vi "tlc_Play.vi"(7 "Reset":bool, 8 "error in (no error)":errorcluster) -> (0 "error out":errorcluster, 3 "Stop?":bool)   [LabVIEW 2010]
doc: "This VI will perform the functionality for playing a Cue for the Theatre Light Controller."
uses:
  Controls/Play.ctl
  Controls/Cue State.ctl
  Modules/Cue/tlc_Cue_Information Command.ctl
  Controls/tlc_User Interface Data Type.ctl
  Modules/Timing/tlc_Timing Command Control.ctl
panel:
  # "Input Data"
  # "Internal Data"
  # "Output Data"
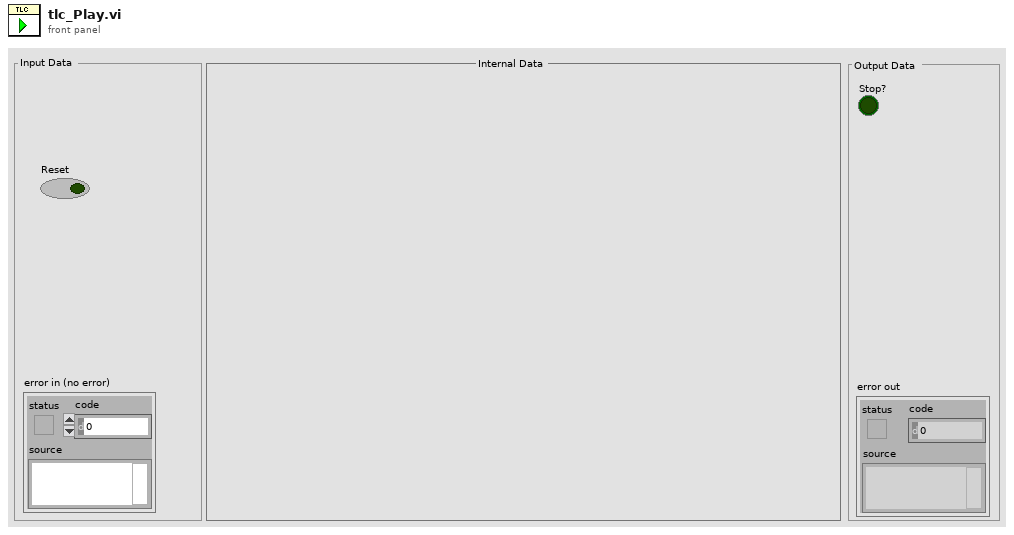
[diagram p1: front panel]
types:
  T1 = typedef "Play.ctl" = enum16{"Initialize", "Begin Play", "Load Cue", "Wait Time", "Fade Time", "Follow Time", "Check for Next Cue", "End Play"}
  T2 = typedef "tlc_Timing Command Control.ctl" = enum16{"Start", "Check Time"}
  T3 = typedef "Cue State.ctl" = cluster{"Desired Intensity":dbl, "Desired Color":u32}
  T4 = typedef "tlc_Cue_Information Command.ctl" = enum16{"Add Cue", "Get Cue Values", "Set Cue Values", "Get Number of Cues", "Initialize", "Get Empty Cue"}
  T5 = typedef "tlc_Cue_Information.ctl" = cluster{"Cue Name":string, "Wait Time (s)":u32, "Fade Time (s)":u32, "Follow Time (s)":u32, "Channels":T6[][]}
  T6 = typedef "channel.ctl" = cluster{"Intensität":dbl, " Farbe":u32, "Channel":i32}
  T7 = typedef "tlc_User Interface Data Type.ctl" = enum16{"Initialize", "Initialize Front Panel", "Update Front Panel Channels", "Select Cue in Cue List", "Enable/Disable Front Panel Controls", "Update Cue List", "Stop"}
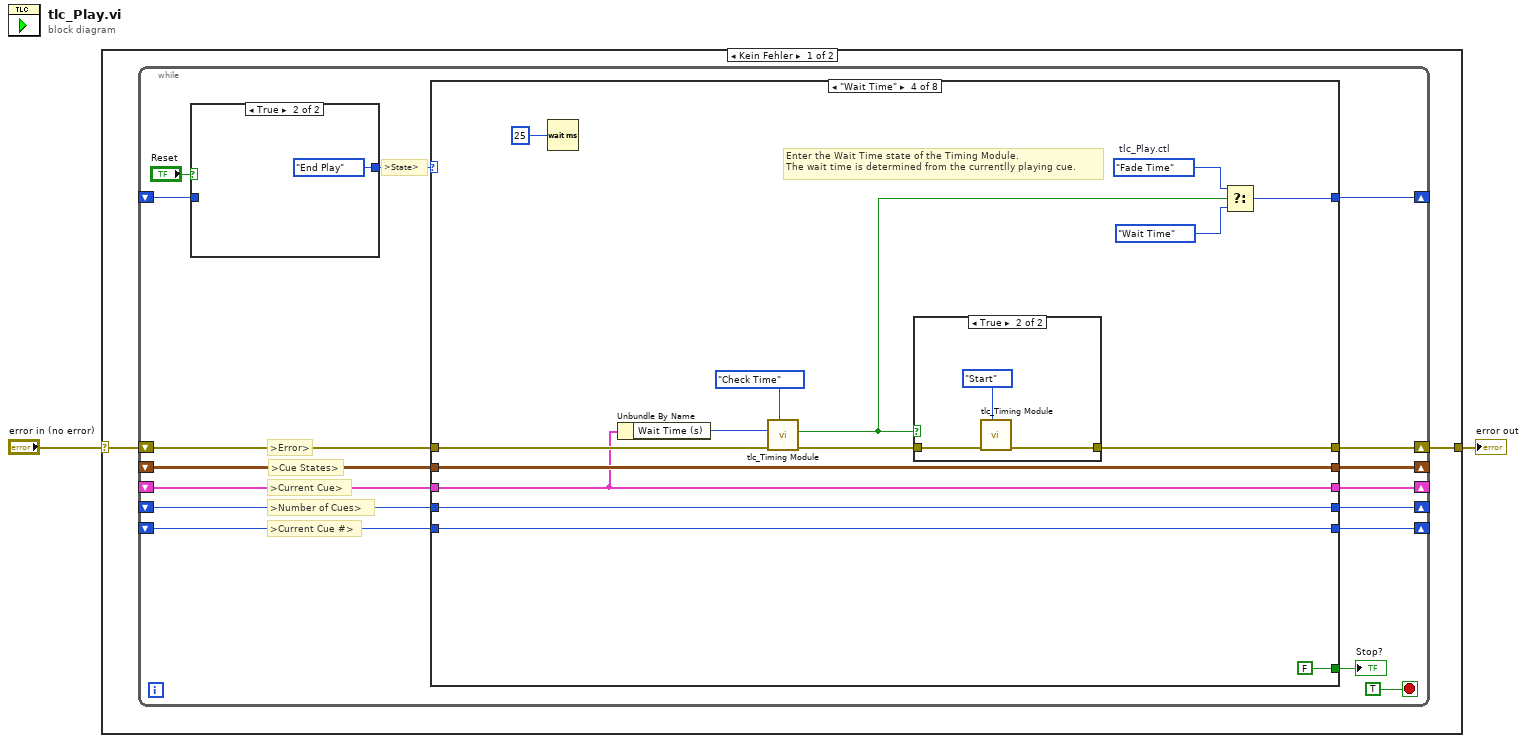
[diagram p0: block diagram]
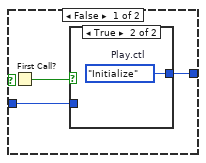
[diagram p2: hidden frame]
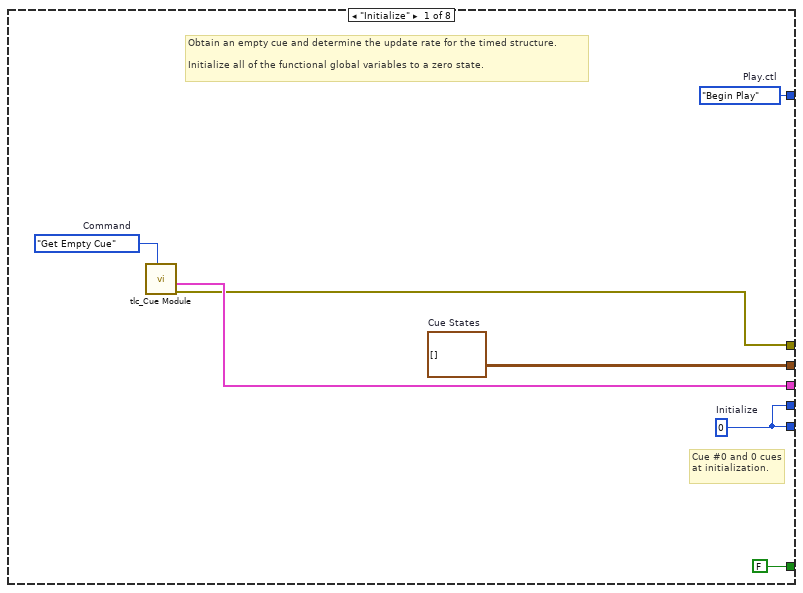
[diagram p4: hidden frame]
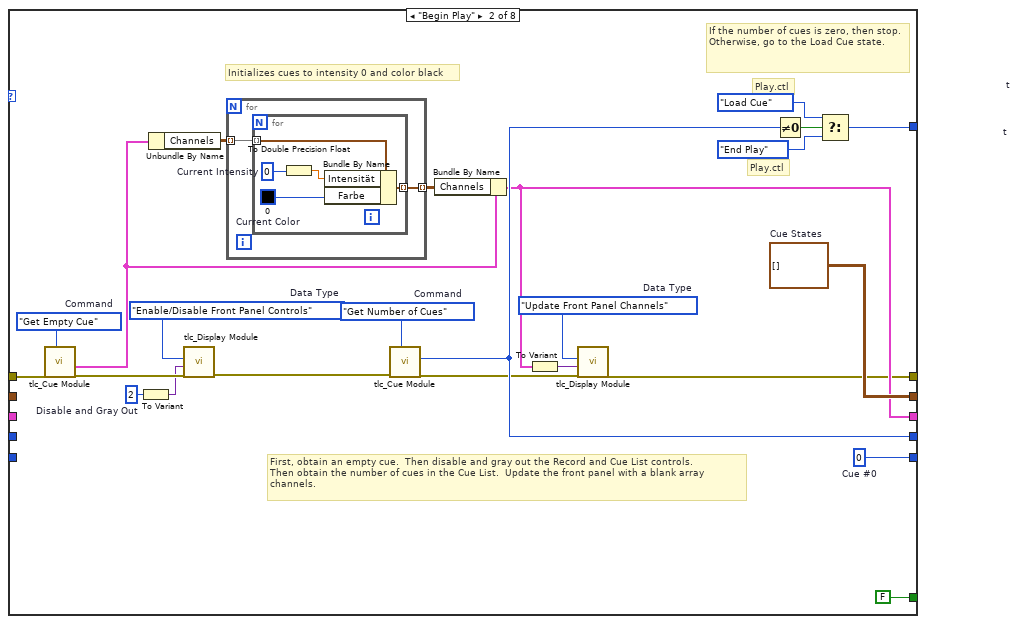
[diagram p5: hidden frame]
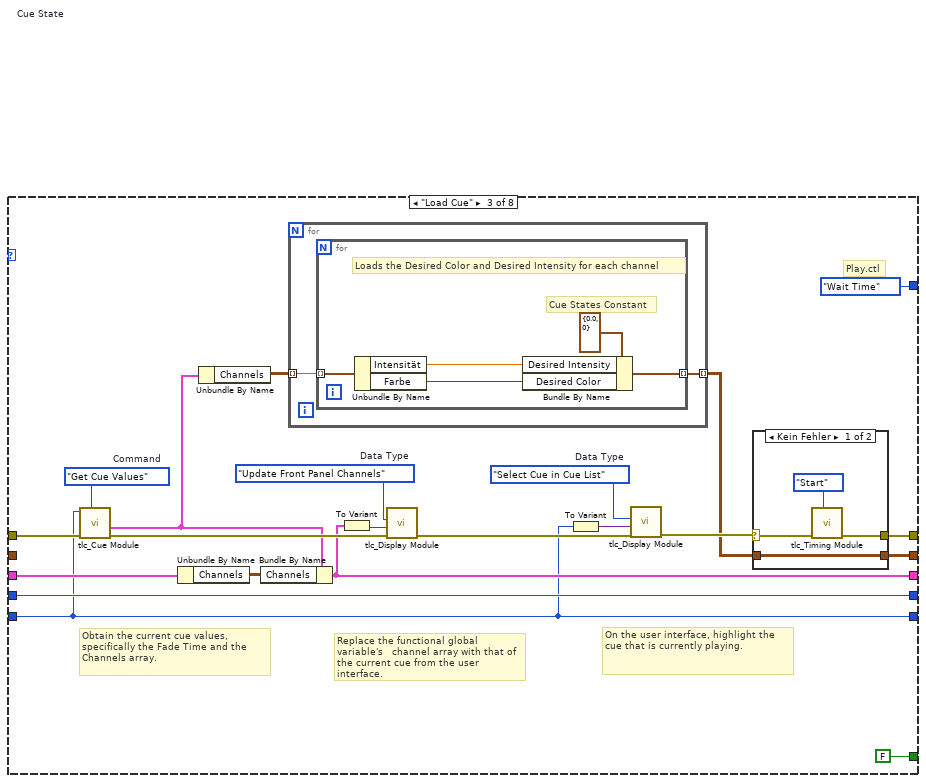
[diagram p6: hidden frame]
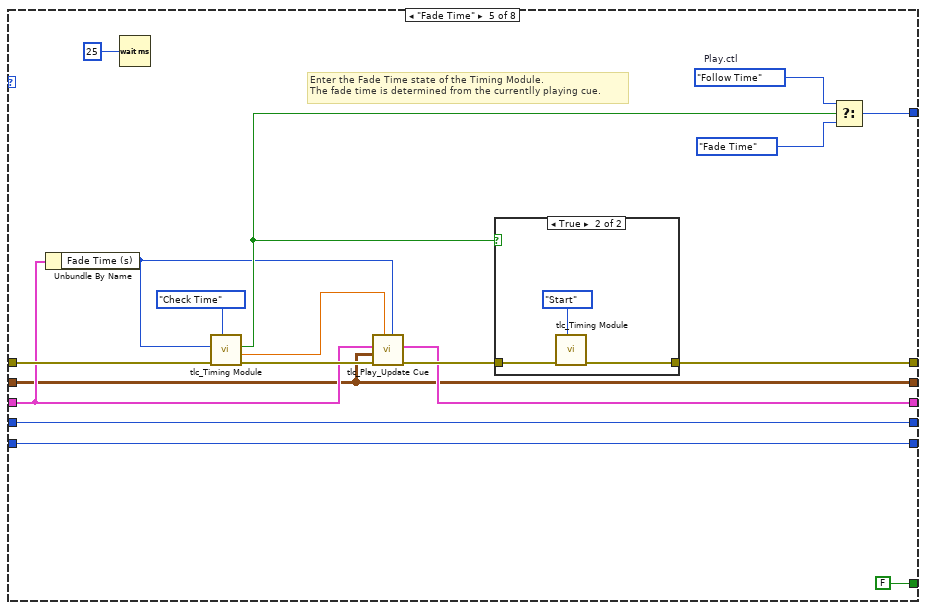
[diagram p9: hidden frame]
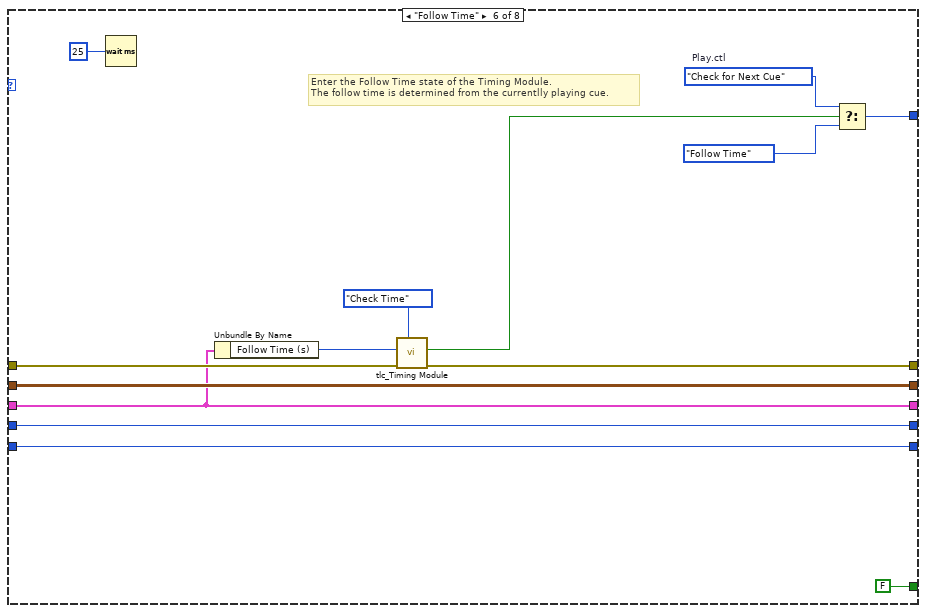
[diagram p11: hidden frame]
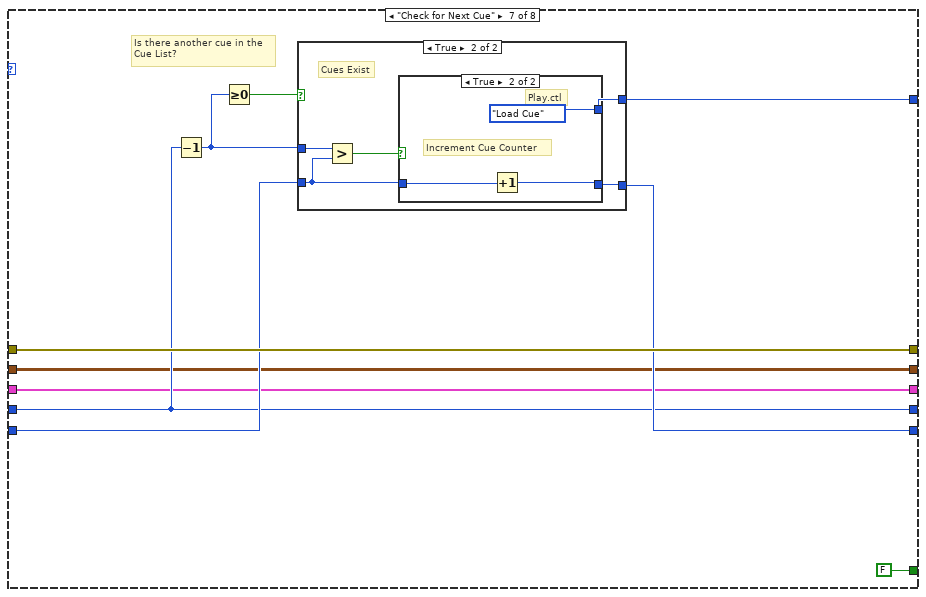
[diagram p12: hidden frame]
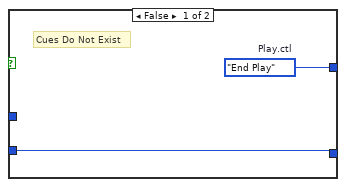
[diagram p13: hidden frame]
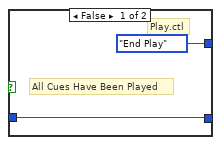
[diagram p14: hidden frame]
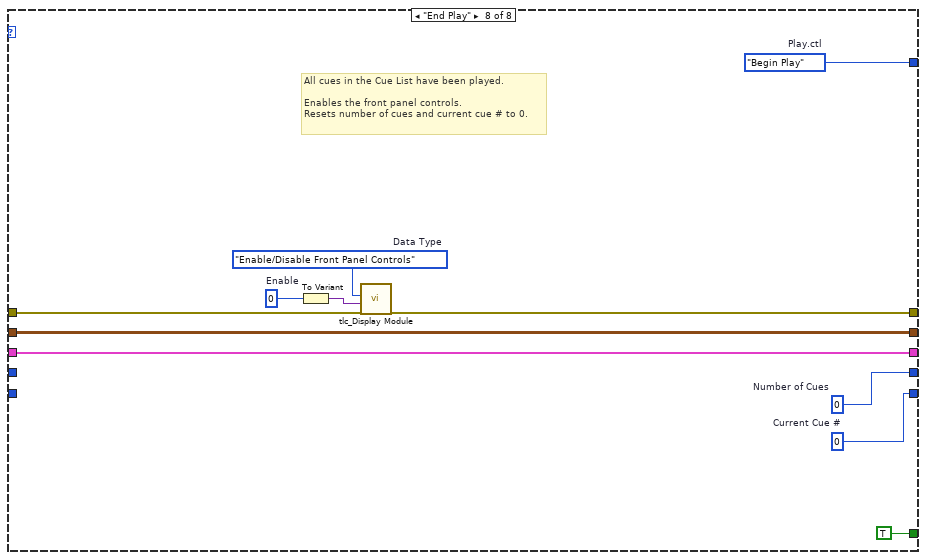
[diagram p15: hidden frame]
diagram:
  n1 = case shown="Kein Fehler" "error in (no error)" {
    selector: "error in (no error)" -> [w3 w187]
    tunnel: [w4 w187] -> w2
    frame No Error {
      n2 = while {
        shift-right: [w19] -> _
        shift-left: _ -> [w8]
        shift-right: [w12] -> w4
        shift-left: w3 -> [w20]
        shift-right: [w18] -> _
        shift-left: _ -> [w17]
        shift-right: [w13] -> _
        shift-left: _ -> [w16]
        shift-right: [w14] -> _
        shift-left: _ -> [w15]
        shift-right: [w7] -> _
        shift-left: _ -> [w6]
        stop <- TRUE stop-if-true
        # ">Cue States>"
        # ">Error>"
        # ">Current Cue #>"
        # ">Number of Cues>"
        # ">State>"
        # ">Current Cue>"
        n3 = case shown="True" "Reset" {
          tunnel: [w23 Play."End Play" ("Play.ctl")] -> w9
          tunnel: w8 -> [w22 _]
          frame False {
            n4 = First Call?() -> (First Call?: T/F=w21:bool)
            n5 = case shown="True" w21 {
              tunnel: [w24 w25] -> w23
              tunnel: w22 -> [w24 _]
              frame False {
              }
              frame True {
                w25 = Play."Initialize"  # Play.ctl
              }
            }
          }
          frame True {
          }
        }
        n6 = case shown="\"Wait Time\"" w9 {
          tunnel: [FALSE FALSE FALSE FALSE FALSE FALSE FALSE TRUE] -> w10
          tunnel: w20 -> [_ w44 w80 w109 w130 w149 w163 w176]
          tunnel: [w27 w34 w67 w104 w132 w145 w163 w180] -> w12
          tunnel: [w32 w54 Play."Wait Time" w103 w128 w144 w160 w186] -> w19
          tunnel: [w33 w45 w73 w113 w135 w153 w156 w183] -> w18
          tunnel: w17 -> [_ _ w73 w113 w135 w153 w156 _]
          tunnel: [w30 w38 w71 w107 w119 w147 w155 w184] -> w13
          tunnel: w16 -> [_ _ w82 w107 w120 w147 w155 w184]
          tunnel: w15 -> [_ _ w70 w112 w134 w152 w158 _]
          tunnel: [w33 w53 w70 w112 w134 w152 w161 w182] -> w14
          tunnel: [w28 w39 w66 w110 w118 w150 w154 w181] -> w7
          tunnel: w6 -> [_ _ _ w110 w118 w150 w154 w181]
          frame "Initialize" {
            w28 = T3[][] []  # Cue States
            w29 = tlc_Cue_Information_Command."Get Empty Cue"  # Command
            w32 = Play."Begin Play"  # Play.ctl
            w33 = 0  # Initialize
            # "Obtain an empty cue and determine the update rate for the timed structure.\n\nInitialize all of the functional global variables to a zero state."
            # "Cue #0 and 0 cues at initialization."
            n7 = call "tlc_Cue Module.vi"("Command"=w29) -> ("error out"=w27:errorcluster, "Cue Output"=w30:T5)  [unwired: 7 in, 1 out]
          }
          frame "Begin Play" {
            w39 = T3[][] []  # Cue States
            w40 = tlc_User_Interface_Data_Type."Update Front Panel Channels"  # Data Type
            w46 = tlc_Cue_Information_Command."Get Number of Cues"  # Command
            w47 = tlc_User_Interface_Data_Type."Enable/Disable Front Panel Controls"  # Data Type
            w48 = tlc_Cue_Information_Command."Get Empty Cue"  # Command
            w55 = Play."End Play"  # t
            w56 = Play."Load Cue"  # t
            w36 = 2  # Disable and Gray Out
            w53 = 0  # Cue #0
            # "Initializes cues to intensity 0 and color black"
            # "If the number of cues is zero, then stop.\nOtherwise, go to the Load Cue state."
            # "First, obtain an empty cue.  Then disable and gray out the Record and Cue List controls.\nThen obtain the number of cues in the Cue List.  Update the front panel with a blank array \nchannels."
            # "Play.ctl"
            # "Play.ctl"
            n8 = call "tlc_Cue Module.vi"("Command"=w48, "error in (no error)"=w44) -> ("error out"=w43:errorcluster, "Cue Output"=w49:T5)  [unwired: 6 in, 1 out]
            n9 = To Variant(anything=w36) -> (Variant=w35:variant)
            n10 = Unbundle By Name(w49) -> ("Channels"=w52:T6[][])
            n11 = call "tlc_Display Module.vi"("error in (no error)"=w43, "Data"=w35, "Data Type"=w47) -> ("error out"=w42:errorcluster)  [unwired: 8 in]
            n12 = for {
              tunnel: w52 -> [w59] mode=indexing
              tunnel: [w58] -> w51 mode=indexing
              n13 = for {
                tunnel: w59 -> [w64] mode=indexing
                tunnel: [w62] -> w58 mode=indexing
                w63 = u32 0  # Current Color
                w61 = u32 0  # Current Intensity
                n14 = To Double Precision Float(number=w61) -> (double precision float=w60:dbl)
                n15 = Bundle By Name(cluster=w64, "Intensität"=w60, "Farbe"=w63) -> (w62:T6)
              }
            }
            n16 = call "tlc_Cue Module.vi"("Command"=w46, "error in (no error)"=w42) -> ("error out"=w41:errorcluster, "Number of Cues"=w45:i32)  [unwired: 6 in, 1 out]
            n17 = Bundle By Name(cluster=w49, "Channels"=w51) -> (w38:T5)
            n18 = To Variant(anything=w38) -> (Variant=w37:variant)
            n19 = call "tlc_Display Module.vi"("error in (no error)"=w41, "Data"=w37, "Data Type"=w40) -> ("error out"=w34:errorcluster)  [unwired: 8 in]
            n20 = Not Equal To 0?(x=w45) -> (x != 0?=w57:bool)
            n21 = Select(t=w56, s=w57, f=w55) -> (s? t:f=w54:T1)
          }
          frame "Load Cue" {
            w74 = tlc_User_Interface_Data_Type."Select Cue in Cue List"  # Data Type
            w76 = tlc_User_Interface_Data_Type."Update Front Panel Channels"  # Data Type
            w78 = tlc_Cue_Information_Command."Get Cue Values"  # Command
            # "On the user interface, highlight the cue that is currently playing."
            # "Replace the functional global variable's   channel array with that of the current cue from the user interface."
            # "Obtain the current cue values, specifically the Fade Time and the Channels array."
            # "Play.ctl"
            n22 = call "tlc_Cue Module.vi"("Command"=w78, "error in (no error)"=w80, "Cue Index"=w70) -> ("error out"=w79:errorcluster, "Cue Output"=w77:T5)  [unwired: 5 in, 1 out]
            n23 = Unbundle By Name(w82) -> ("Channels"=w81:T6[][])
            n24 = Unbundle By Name(w77) -> ("Channels"=w84:T6[][])
            n25 = Bundle By Name(cluster=w77, "Channels"=w81) -> (w71:T5)
            n26 = for {
              tunnel: w84 -> [w93] mode=indexing
              tunnel: [w92] -> w65 mode=indexing
              n27 = for {
                tunnel: w93 -> [w98] mode=indexing
                tunnel: [w96] -> w92 mode=indexing
                w95 = T3 {"Desired Intensity"=0.0, "Desired Color"=0}  # Cue State
                # "Loads the Desired Color and Desired Intensity for each channel"
                # "Cue States Constant"
                n28 = Unbundle By Name(w98) -> ("Intensität"=w94:dbl, "Farbe"=w97:u32)
                n29 = Bundle By Name(cluster=w95, "Desired Intensity"=w94, "Desired Color"=w97) -> (w96:T3)
              }
            }
            n30 = To Variant(anything=w71) -> (Variant=w72:variant)
            n31 = call "tlc_Display Module.vi"("error in (no error)"=w79, "Data"=w72, "Data Type"=w76) -> ("error out"=w75:errorcluster)  [unwired: 8 in]
            n32 = To Variant(anything=w70) -> (Variant=w69:variant)
            n33 = call "tlc_Display Module.vi"("error in (no error)"=w75, "Data"=w69, "Data Type"=w74) -> ("error out"=w68:errorcluster)  [unwired: 8 in]
            n34 = case shown="Kein Fehler" w68 {
              selector: w68 -> [w88 w91]
              tunnel: [w87 w91] -> w67
              tunnel: [w89 w90] -> w66
              tunnel: w65 -> [w89 w90]
              frame No Error {
                n35 = call "tlc_Timing Module.vi"("Kommando"=tlc_Timing_Command_Control."Start" ("Timer Command"), "error in (no error)"=w88) -> ("error out"=w87:errorcluster)  [unwired: 7 in, 2 out]
              }
              frame Error {
              }
            }
          }
          frame "Wait Time" {
            w102 = Play."Fade Time"  # tlc_Play.ctl
            # "Enter the Wait Time state of the Timing Module.\nThe wait time is determined from the currentlly playing cue."
            n36 = Wait (ms)(milliseconds to wait=u32 25) -> ()  [unwired: 1 out]
            n37 = Unbundle By Name "Unbundle By Name"(w107) -> ("Wait Time (s)"=w106:u32)
            n38 = call "tlc_Timing Module.vi"("Kommando"=tlc_Timing_Command_Control."Check Time" ("Command"), "error in (no error)"=w109, "Ziel Zeit"=w106) -> ("error out"=w105:errorcluster, "Fertig?"=w100:bool)  [unwired: 6 in, 1 out]
            n39 = case shown="True" w100 {
              tunnel: w105 -> [w114 w117]
              tunnel: [w114 w116] -> w104
              frame False {
              }
              frame True {
                n40 = call "tlc_Timing Module.vi"("Kommando"=tlc_Timing_Command_Control."Start" ("Timer Command"), "error in (no error)"=w117) -> ("error out"=w116:errorcluster)  [unwired: 7 in, 2 out]
              }
            }
            n41 = Select(t=w102, s=w100, f=Play."Wait Time" ("t")) -> (s? t:f=w103:T1)
          }
          frame "Fade Time" {
            w126 = Play."Follow Time"  # Play.ctl
            # "Enter the Fade Time state of the Timing Module.\nThe fade time is determined from the currentlly playing cue."
            n42 = Unbundle By Name "Unbundle By Name"(w120) -> ("Fade Time (s)"=w121:u32)
            n43 = Wait (ms)(milliseconds to wait=u32 25) -> ()  [unwired: 1 out]
            n44 = call "tlc_Timing Module.vi"("Kommando"=tlc_Timing_Command_Control."Check Time" ("Timer Command"), "error in (no error)"=w130, "Ziel Zeit"=w121) -> ("error out"=w124:errorcluster, "Verstrichene Zeit"=w122:dbl, "Fertig?"=w125:bool)  [unwired: 6 in]
            n45 = call "tlc_Play_Update Cue.vi"("Target Time"=w121, "Elapsed Time"=w122, "error in"=w124, "Cue States"=w118, "Cue Input"=w120) -> ("error out"=w123:errorcluster, "Cue Output"=w119:T5)  [unwired: 5 in]
            n46 = case shown="True" w125 {
              tunnel: [w136 w139] -> w132
              tunnel: w123 -> [w136 w137]
              frame False {
              }
              frame True {
                n47 = call "tlc_Timing Module.vi"("Kommando"=tlc_Timing_Command_Control."Start" ("Command"), "error in (no error)"=w137) -> ("error out"=w139:errorcluster)  [unwired: 7 in, 2 out]
              }
            }
            n48 = Select(t=w126, s=w125, f=Play."Fade Time") -> (s? t:f=w128:T1)
          }
          frame "Follow Time" {
            w143 = Play."Check for Next Cue"  # Play.ctl
            # "Enter the Follow Time state of the Timing Module.\nThe follow time is determined from the currentlly playing cue."
            n49 = Wait (ms)(milliseconds to wait=u32 25) -> ()  [unwired: 1 out]
            n50 = Unbundle By Name "Unbundle By Name"(w147) -> ("Follow Time (s)"=w146:u32)
            n51 = call "tlc_Timing Module.vi"("Kommando"=tlc_Timing_Command_Control."Check Time" ("Command"), "error in (no error)"=w149, "Ziel Zeit"=w146) -> ("error out"=w145:errorcluster, "Fertig?"=w141:bool)  [unwired: 6 in, 1 out]
            n52 = Select(t=w143, s=w141, f=Play."Follow Time") -> (s? t:f=w144:T1)
          }
          frame "Check for Next Cue" {
            # "Is there another cue in the \nCue List?"
            n53 = Decrement(x=w156) -> (x-1=w157:i32)
            n54 = Greater Or Equal To 0?(x=w157) -> (x >= 0?=w159:bool)
            n55 = case shown="True" w159 {
              tunnel: [w165 w170] -> w161
              tunnel: [w164 w169] -> w160
              tunnel: w158 -> [w165 w166]
              tunnel: w157 -> [_ w167]
              frame False {
                w164 = Play."End Play"  # Play.ctl
                # "Cues Do Not Exist"
              }
              frame True {
                # "Cues Exist"
                n56 = Greater?(x=w167, y=w166) -> (0:w168:bool)
                n57 = case shown="True" w168 {
                  tunnel: w166 -> [w171 w175]
                  tunnel: [w171 w174] -> w170
                  tunnel: [Play."End Play" ("t") Play."Load Cue" ("t")] -> w169
                  frame False {
                    # "Play.ctl"
                    # "All Cues Have Been Played"
                  }
                  frame True {
                    # "Play.ctl"
                    # "Increment Cue Counter"
                    n58 = Increment(x=w175) -> (x+1=w174:i32)
                  }
                }
              }
            }
          }
          frame "End Play" {
            w179 = tlc_User_Interface_Data_Type."Enable/Disable Front Panel Controls"  # Data Type
            w186 = Play."Begin Play"  # Play.ctl
            w178 = 0  # Enable
            w182 = 0  # Current Cue #
            w183 = 0  # Number of Cues
            # "All cues in the Cue List have been played.\n\nEnables the front panel controls.\nResets number of cues and current cue # to 0."
            n59 = To Variant(anything=w178) -> (Variant=w177:variant)
            n60 = call "tlc_Display Module.vi"("error in (no error)"=w176, "Data"=w177, "Data Type"=w179) -> ("error out"=w180:errorcluster)  [unwired: 8 in]
          }
        }
        "Stop?" <- w10
      }
    }
    frame Error {
    }
  }
  "error out" <- w2
